vi "ToRepo.vi"(8 "error in":errorcluster, 9 "to repo cluster":T1, 10 "repository in":refnum<class "CEF_Repository.lvclass">, 11 "CEF_Node in":refnum<class "CEF_Node.lvclass">) -> (0 "error out":errorcluster, 2 "repository out":refnum<class "CEF_Repository.lvclass">, 3 "CEF_Node out":refnum<class "CEF_Node.lvclass">)   [LabVIEW 2025, in "CEF.lvlib" / "CEF_Node.lvclass"]
doc: "Transfers the information from the tree node into the repo. How it is stored in the repo depends on the Repo.Copyright 2017 National Instruments Corporation\n\nLicensed under the Apache License, Version 2.0 (the \"License\"); you may not use this file except in compliance with the License. You may obtain a copy of the License at http://www.apache.org/licenses/LICENSE-2.0\nUnless required by applicable law or agreed to in writing, software distributed under the License is distributed on an \"AS IS\" BASIS, WITHOUT WARRANTIES OR CONDITIONS OF ANY KIND, either express or implied. See the License for the specific language governing permissions and limitations under the License."
uses:
  CEF_Node.lvclass
  Repository/CEF_Repository.lvclass
  ToRepoCluster.ctl
  CEF_Node.lvclass/CEF_Node.ctl
  ReadChildren.vi
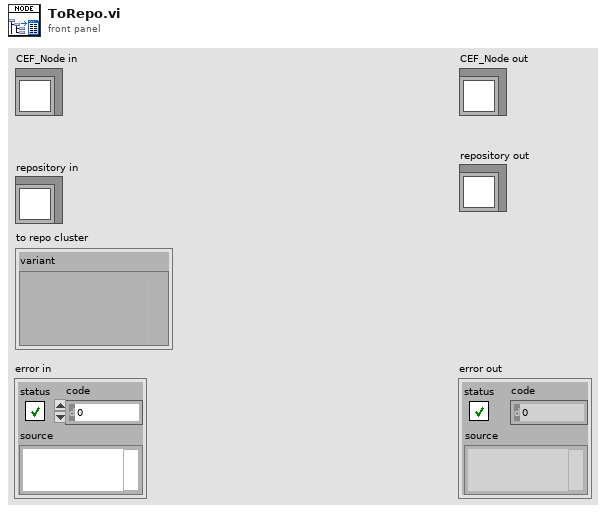
[diagram p1: front panel]
types:
  T1 = typedef "CEF.lvlib/CEF_Node.lvclass/ToRepoCluster.ctl" = cluster{"variant":variant}
  T2 = typedef "CEF.lvlib/CEF_Node.lvclass/NodeRef.ctl" = refnum<data-value>
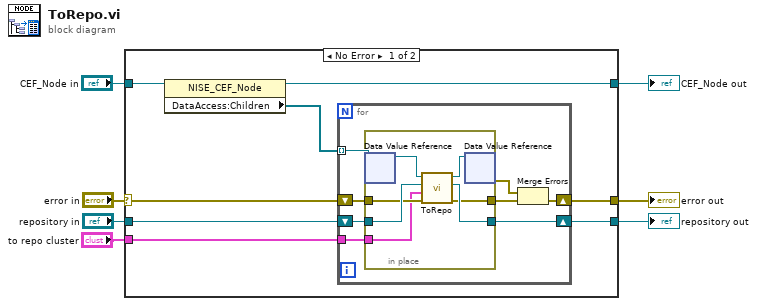
[diagram p0: block diagram]
diagram:
  n1 = case shown="No Error" "error in" {
    selector: "error in" -> [w11 w33]
    tunnel: [w10 w33] -> w6
    tunnel: [w9 w32] -> w4
    tunnel: "CEF_Node in" -> [w15 w32]
    tunnel: "repository in" -> [w13 w31]
    tunnel: [w12 w31] -> w2
    tunnel: "to repo cluster" -> [w8 _]
    frame No Error {
      n2 = property class="NISE_CEF_Node"(reference=w15) -> (reference out=w9:refnum<class "CEF_Node.lvclass">, "DataAccess:Children"=w14:T2[])  [unwired: 1 in, 1 out]
      n3 = for {
        tunnel: w14 -> [w23] mode=indexing
        shift-right: [w21] -> w12
        shift-left: w13 -> [w22]
        shift-right: [w17] -> w10
        shift-left: w11 -> [w20]
        tunnel: w8 -> [w19]
        n4 = in-place {
          in-place-border: w22 -> [w29]
          in-place-border: [w28] -> w21
          in-place-border: w20 -> [w27]
          in-place-border: [w26] -> w18
          in-place-border: w19 -> [w24]
          n5 = in-place-dvr #1(w23) -> (w30:refnum<class "CEF_Node.lvclass">)  [unwired: 1 out]
          n6 = call-dynamic "ToRepo.vi"("error in"=w27, "to repo cluster"=w24, "repository in"=w29, "CEF_Node in"=w30) -> ("error out"=w26:errorcluster, "repository out"=w28:refnum<class "CEF_Repository.lvclass">, "CEF_Node out"=w25:refnum<class "CEF_Node.lvclass">)  [unwired: 5 in]
          n7 = in-place-dvr #1(w25) -> (w16:errorcluster)  [unwired: 1 out]
        }
        n8 = Merge Errors(w16, w18) -> (w17:errorcluster)
      }
    }
    frame Error {
    }
  }
  "error out" <- w6
  "CEF_Node out" <- w4
  "repository out" <- w2
